vi "mapping.vi"(0 "max out":dbl, 2 "min out":dbl, 3 "max in":dbl, 4 "in":dbl, 5 "min in":dbl) -> (1 "out":dbl)   [LabVIEW 2018]
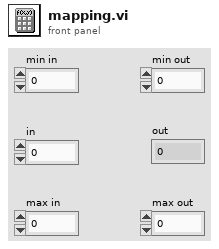
[diagram p1: front panel]
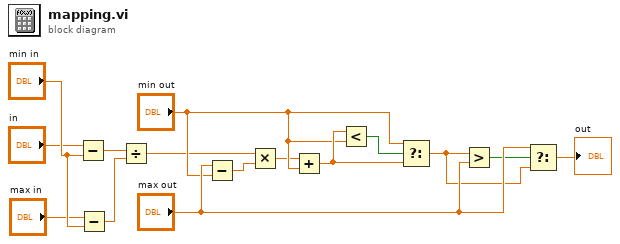
[diagram p0: block diagram]
diagram:
  n1 = Subtract(x="in", y="min in") -> (x-y=w4:dbl)
  n2 = Subtract(x="max in", y="min in") -> (x-y=w5:dbl)
  n3 = Divide(x=w4, y=w5) -> (x/y=w6:dbl)
  n4 = Subtract(x="max out", y="min out") -> (x-y=w7:dbl)
  n5 = Multiply(x=w6, y=w7) -> (x*y=w8:dbl)
  n6 = Add(x=w8, y="min out") -> (x+y=w11:dbl)
  n7 = Less?(x=w11, y="min out") -> (x < y?=w9:bool)
  n8 = Select(t="min out", s=w9, f=w11) -> (s? t:f=w12:dbl)
  n9 = Greater?(x=w12, y="max out") -> (0:w13:bool)
  n10 = Select(t="max out", s=w13, f=w12) -> (s? t:f=→"out":dbl)
